vi "ReadMatrix.vi"(9 "byte order":T3(ring)=enum."little-endian", 11 "String in":string) -> (0 "Data":T4, 1 "Class":T5(ring), 2 "Dimensions":u32[](array[numeric]), 3 "Matrix":T2)   [LabVIEW 2022 SP3]
uses:
  miDataType.ctl
panel:
  out "data":string
  out "length":i32
  out "String out":string
  out "Waveform Graph":dbl[][](graph)
  out "value":dbl[](array[numeric]) format="%.6f"
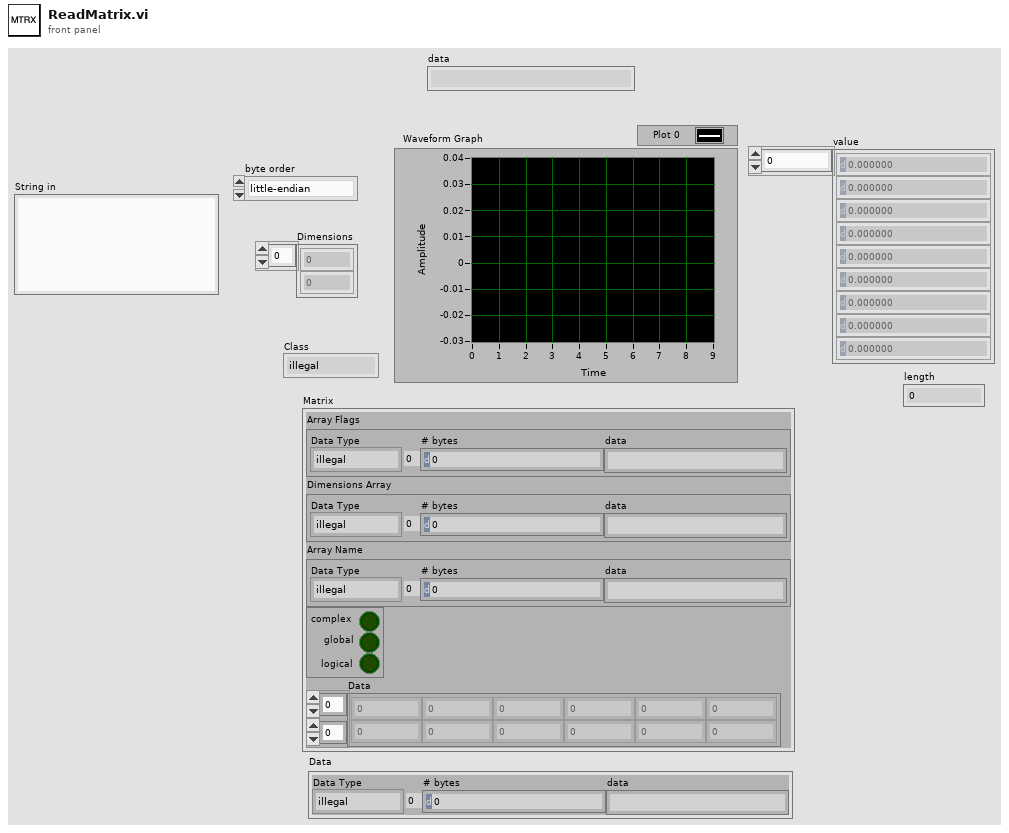
[diagram p1: front panel]
types:
  T1 = typedef "miDataType.ctl" = enum16{"illegal", "miINT8", "miUINT8", "miINT16", "miUINT16", "miINT32", "miUINT32", "miSINGLE", "--", "miDOUBLE", "---", "----", "miINT64", "miUINT64", "miMATRIX", "miCOMPRESSED", "miUTF8", "miUTF16", "miUTF32", "udefined"}
  T2 = cluster{"Array Flags":cluster{"Data Type":T1, "# bytes":u32, "data":string}, "Dimensions Array":cluster{"Data Type":T1, "# bytes":u32, "data":string}, "Array Name":cluster{"Data Type":T1, "# bytes":u32, "data":string}, cluster{"complex":bool, "global":bool, "logical":bool}, "Data":dbl[][]}
  T3 = enum16{"big-endian, network order", "native, host order", "little-endian"}
  T4 = cluster{"Data Type":T1, "# bytes":u32, "data":string}
  T5 = enum16{"illegal", "Cell array", "Structure", "Object", "Character Array", "Sparse Array", "Double Array", "Single Array", "i8", "u8", "i16", "u16", "i32", "u32", "i64", "u64"}
  T6 = cluster{"Tag":cluster{"Data Type":T1, "# bytes":u32, "data":string}, "Tag":cluster{"Data Type":T1, "# bytes":u32, "data":string}, "Tag":cluster{"Data Type":T1, "# bytes":u32, "data":string}, cluster{bool, bool, bool}, dbl[][]}
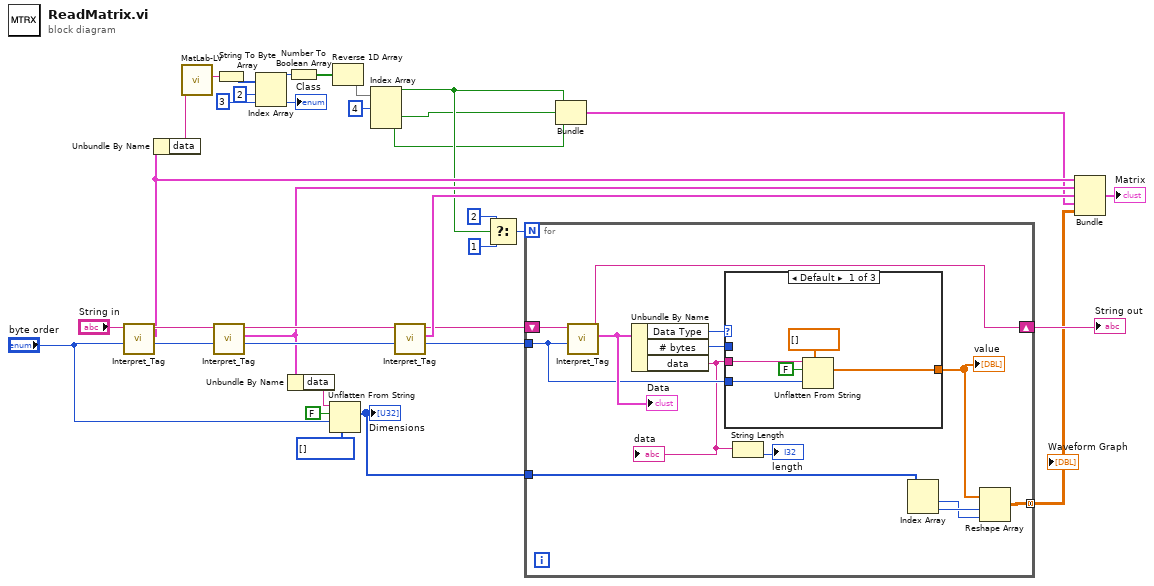
[diagram p0: block diagram]
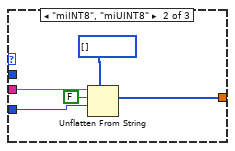
[diagram p2: hidden frame]
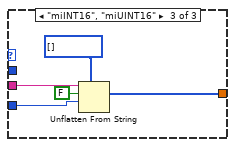
[diagram p3: hidden frame]
diagram:
  n1 = call "Interpret_Tag.vi"("byte order"="byte order", "String in"="String in") -> ("Tag"=w13:T4, "String out"=w19:string)  [unwired: 7 in, 1 out]
  n2 = Unbundle By Name(w13) -> ("data"=w1:string)
  n3 = call "MatLab-LV.vi"("data in"=w1) -> ("data out"=w29:string)  [unwired: 10 in]
  n4 = call "Interpret_Tag.vi"("byte order"="byte order", "String in"=w19) -> ("Tag"=w12:T4, "String out"=w20:string)  [unwired: 7 in, 1 out]
  n5 = String To Byte Array(string=w29) -> (unsigned byte array=w21:u8[])
  n6 = Index Array(array=w21, index #1=2 ("index"), index #2=3 ("index")) -> (element #1=w24:u8, element #2=→"Class":u8)
  n7 = Unbundle By Name(w12) -> ("data"=w17:string)
  n8 = Number To Boolean Array(number=w24) -> (Boolean array=w25:bool[])
  n9 = Unflatten From String(type=u32[] [], binary string=w17, data includes array or string size? (T)=FALSE, byte order (0:big-endian, network order)="byte order") -> (value=w32:u32[])  [unwired: 1 in, 2 out]
  "Dimensions" <- w32
  n10 = Reverse 1D Array(array=w25) -> (reversed array=w28:bool[])
  n11 = Index Array(array=w28, index #1=4 ("index")) -> (element #1=w10:bool, element #2=w9:bool, element #3=w8:bool)  [unwired: 2 in]
  n12 = call "Interpret_Tag.vi"("byte order"="byte order", "String in"=w20) -> ("Tag"=w11:T4, "String out"=w3:string)  [unwired: 7 in, 1 out]
  n13 = Select(t=2, s=w10, f=1) -> (s? t:f=w2:i32)
  n14 = for {
    N: w2 -> [_]
    tunnel: w32 -> [w43]
    tunnel: [w39] -> w6 mode=concatenating
    shift-right: [w35] -> w14
    shift-left: w3 -> [w37]
    tunnel: "byte order" -> [w36]
    n15 = call "Interpret_Tag.vi"("byte order"=w36, "String in"=w37) -> ("Tag"=w42:T4, "String out"=w35:string)  [unwired: 7 in, 1 out]
    "Data" <- w42
    n16 = Unbundle By Name(w42) -> ("Data Type"=w41:T1, "# bytes"=w40:u32, "data"=w33:string)
    "data" <- w33
    n17 = case shown="Default" w41 {
      tunnel: w40 -> [_ _ _]
      tunnel: w33 -> [w48 w54 w59]
      tunnel: [w47 w52 w57] -> w38
      tunnel: w36 -> [w46 w51 w56]
      frame Default {
        n18 = Unflatten From String(type=dbl[] [], binary string=w48, data includes array or string size? (T)=FALSE, byte order (0:big-endian, network order)=w46) -> (value=w47:dbl[])  [unwired: 1 in, 2 out]
      }
      frame "miINT8", "miUINT8" {
        n19 = Unflatten From String(type=u8[] [], binary string=w54, data includes array or string size? (T)=FALSE, byte order (0:big-endian, network order)=w51) -> (value=w52:u8[])  [unwired: 1 in, 2 out]
      }
      frame "miINT16", "miUINT16" {
        n20 = Unflatten From String(type=u16[] [], binary string=w59, data includes array or string size? (T)=FALSE, byte order (0:big-endian, network order)=w56) -> (value=w57:u16[])  [unwired: 1 in, 2 out]
      }
    }
    "value" <- w38
    n21 = String Length(string=w33) -> (length=→"length":i32)
    n22 = Index Array(array=w43) -> (element #1=w44:u32, element #2=w45:u32)  [unwired: 2 in]
    n23 = Reshape Array(w38, w45, w44) -> (w39:dbl[][])
  }
  "Waveform Graph" <- w6
  "String out" <- w14
  n24 = Bundle(w10, w9, w8) -> (w7:cluster{bool, bool, bool})  [unwired: 1 in]
  n25 = Bundle("Tag"=w13, "Tag"=w12, "Tag"=w11, w7, w6) -> (→"Matrix":T6)  [unwired: 1 in]
